vi "Min-SP-UpdateChannels.vi"(8 "Error In":errorcluster, 10 "CD Settings In":T1={"CD Task Dependency"=18446744073709551615, "CD Task Dependency Ref"=18446744073709551615, "CD Task Available Wfms"=[], "CD Task Selected Wfms"=[], "Buffer Length (samples)"=0, "Min Enabled"=FALSE, "Max Enabled "=FALSE, "SP Enabled"=FALSE, "RMS Enabled"=FALSE, "Buffer Length (s)"=0.0, "Task Rate"=0.0, "Number of DAQ Chanels"=0} {"CD Task Dependency Ref" format="%.0x"; "CD Task Dependency" format="%.0x"}, 11 "Item Ref in":T2 format="%.0x") -> (0 "Error Out":errorcluster, 2 "CD Settings Out":T1={"CD Task Dependency"=18446744073709551615, "CD Task Dependency Ref"=18446744073709551615, "CD Task Available Wfms"=[], "CD Task Selected Wfms"=[], "Buffer Length (samples)"=0, "Min Enabled"=FALSE, "Max Enabled "=FALSE, "SP Enabled"=FALSE, "RMS Enabled"=FALSE, "Buffer Length (s)"=0.0, "Task Rate"=0.0, "Number of DAQ Chanels"=0} {"CD Task Dependency Ref" format="%.0x"; "CD Task Dependency" format="%.0x"}, 3 "Item Ref Out":T2=18446744073709551615 format="%.0x")   [LabVIEW 2017, in "Waveform-Processing-Custom-Device Shared.lvlib" / "Min_SP.lvlib"]
uses:
  Min_SP.lvlib
  <vilib>/NI Veristand/Custom Device API/Custom Device Item Ref.ctl
  Custom Device Settings.ctl
  <vilib>/NI VeriStand/Custom Device API/Custom Device API.lvlib
  Waveform-Processing-Custom-Device Shared.lvlib
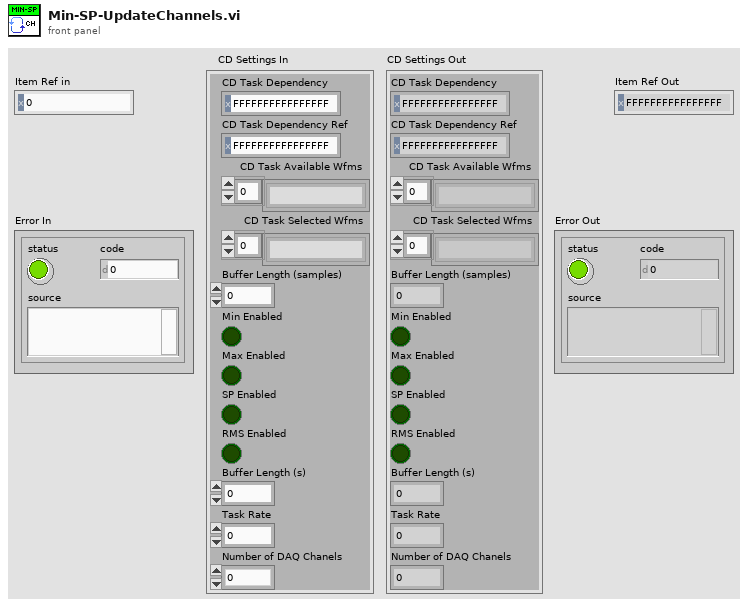
[diagram p1: front panel]
types:
  T1 = typedef "Waveform-Processing-Custom-Device Shared.lvlib/Custom Device Settings.ctl" = cluster{"CD Task Dependency":T2, "CD Task Dependency Ref":T2, "CD Task Available Wfms":string[], "CD Task Selected Wfms":string[], "Buffer Length (samples)":u32, "Min Enabled":bool, "Max Enabled ":bool, "SP Enabled":bool, "RMS Enabled":bool, "Buffer Length (s)":dbl, "Task Rate":dbl, "Number of DAQ Chanels":u32}
  T2 = typedef "Custom Device API.lvlib/Custom Device Item Ref.ctl" = u64
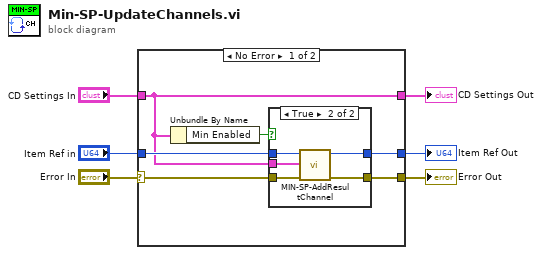
[diagram p0: block diagram]
diagram:
  n1 = case shown="No Error" "Error In" {
    selector: "Error In" -> [w9 w22]
    tunnel: [w12 w22] -> w3
    tunnel: "Item Ref in" -> [w10 w21]
    tunnel: [w11 w21] -> w4
    tunnel: [w7 w20] -> w2
    tunnel: "CD Settings In" -> [w7 w20]
    frame No Error {
      n2 = Unbundle By Name(w7) -> ("Min Enabled"=w8:bool)
      n3 = case shown="True" w8 {
        tunnel: w9 -> [w13 w18]
        tunnel: [w13 w16] -> w12
        tunnel: w10 -> [w14 w19]
        tunnel: [w14 w17] -> w11
        tunnel: w7 -> [_ w15]
        frame False {
        }
        frame True {
          n4 = call "MIN-SP-AddResultChannel.vi"("Error In"=w18, "CD Settings"=w15, "Device Ref in"=w19) -> ("Error Out"=w16:errorcluster, "Device Ref Out"=w17:T2)  [unwired: 7 in]
        }
      }
    }
    frame Error {
    }
  }
  "Error Out" <- w3
  "Item Ref Out" <- w4
  "CD Settings Out" <- w2
